vi "SetTestStatus.vi"(0 "reference in":refnum<class "Test.lvclass">, 1 "Test Status":T1(ring), 5 "error in (no error)":errorcluster) -> (14 "reference out":refnum<class "Test.lvclass">, 19 "error out":errorcluster)   [LabVIEW 2024, in "Test.lvclass"]
uses:
  Test.lvclass
  Test.lvclass/Test.ctl
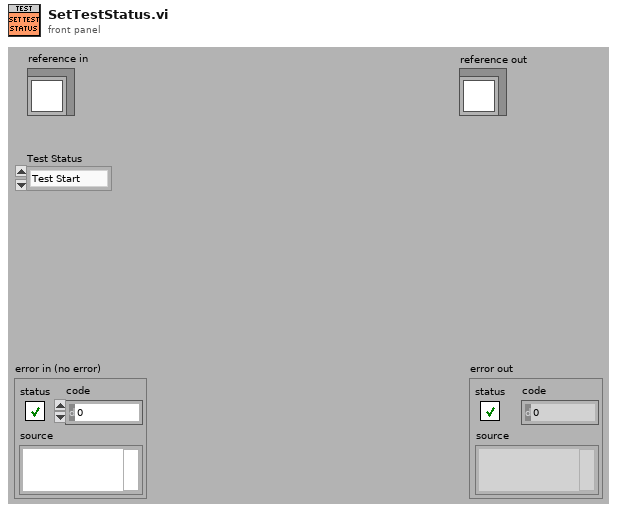
[diagram p1: front panel]
types:
  T1 = enum16{"Test Start", "Test Continue", "Test Failed", "Test Success"}
  T2 = typedef "Test.lvclass/ObjectAttributes.ctl" = cluster{"Engine":bool, "Dynamometer":bool, "Test Status":enum16{"Test Start", "Test Continue", "Test Failed", "Test Success"}, "History String":string}
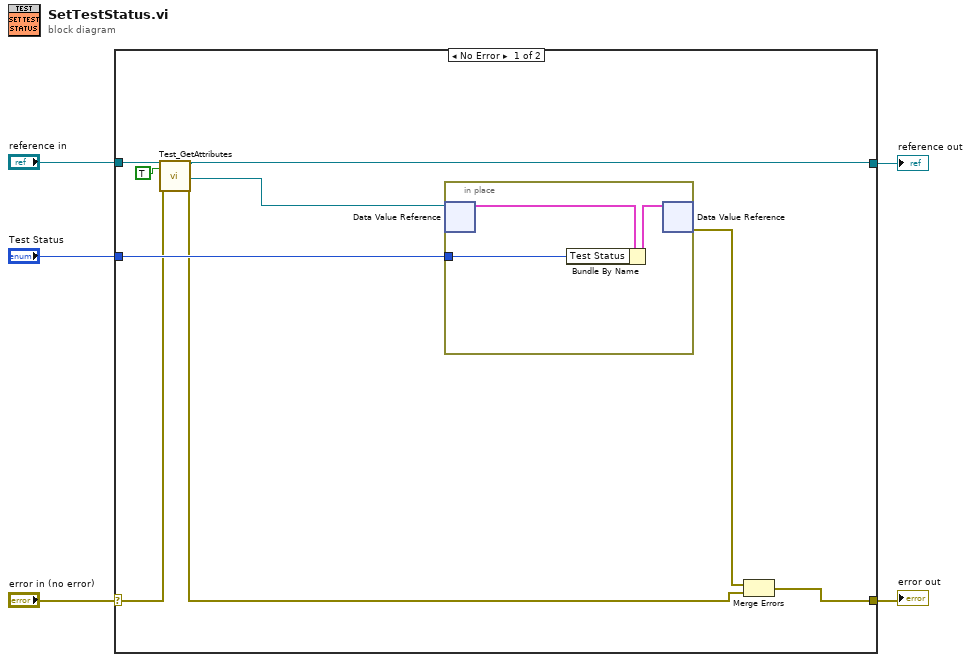
[diagram p0: block diagram]
diagram:
  n1 = case shown="No Error" "error in (no error)" {
    selector: "error in (no error)" -> [w8 w19]
    tunnel: [w12 w19] -> w4
    tunnel: [w10 w18] -> w2
    tunnel: "reference in" -> [w11 w18]
    tunnel: "Test Status" -> [w14 _]
    frame No Error {
      n2 = call "Test_GetAttributes.vi"("reference in"=w11, "OnlyGetDvrReference(False)"=TRUE, "error in (no error)"=w8) -> ("reference out"=w10:refnum<class "Test.lvclass">, "DataRef"=w9:refnum<data-value>, "error out"=w7:errorcluster)  [unwired: 13 in, 1 out]
      n3 = in-place {
        in-place-border: w14 -> [w17]
        n4 = in-place-dvr #1(w9) -> (w16:T2)  [unwired: 1 out]
        n5 = Bundle By Name(cluster=w16, "Test Status"=w17) -> (w15:T2)
        n6 = in-place-dvr #1(w15) -> (w13:errorcluster)  [unwired: 1 out]
      }
      n7 = Merge Errors(w13, w7) -> (w12:errorcluster)
    }
    frame Error {
    }
  }
  "error out" <- w4
  "reference out" <- w2
